vi "DataLog Append Meta Specifier.vi"(0 "meta specifier":T1, 7 "tag in":string) -> (8 "tag out":string)   [LabVIEW 2012]
doc: "This VI appends one of the meta specifiers to a tag so as to obtain the name of the corresponding meta tag. If \"not a meta\" is specified, the input tag is returned. This VI is the inverse of \"Strip Meta Specifier\"."
uses:
  typedefs/et_DataLog Meta Tag Specifier.ctl
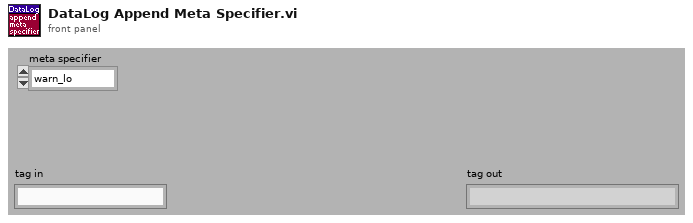
[diagram p1: front panel]
types:
  T1 = typedef "et_DataLog Meta Tag Specifier.ctl" = enum32{"warn_lo", "warn_hi", "A_lo", "A_hi", "B_lo", "B_hi", "C_lo", "C_hi", "D_lo", "D_hi", "E_lo", "E_hi", "F_lo", "F_hi", "G_lo", "G_hi", "H_lo", "H_hi", "I_lo", "I_hi", "J_lo", "J_hi", "K_lo", "K_hi", "L_lo", "L_hi", "M_lo", "M_hi", "N_lo", "N_hi", "min", "max", "not a meta"}
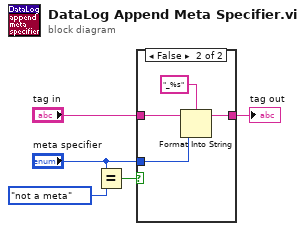
[diagram p0: block diagram]
diagram:
  n1 = Equal?(x="meta specifier", y=et_DataLog_Meta_Tag_Specifier."not a meta" ("meta specifier")) -> (x = y?=w1:bool)
  n2 = case shown="False" w1 {
    tunnel: "tag in" -> [w6 w9]
    tunnel: [w6 w8] -> w5
    tunnel: "meta specifier" -> [_ w7]
    frame True {
    }
    frame False {
      n3 = Format Into String(format string="_%s", initial string=w9, w7) -> (resulting string=w8:string)  [unwired: 1 in, 1 out]
    }
  }
  "tag out" <- w5
